vi "Ballard 1553 - Initialization VI.vi"(8 "error in (no error)":errorcluster, 10 "Custom XML":string, 11 "Device Item Ref in":T1 format="%.0x") -> (0 "error out":errorcluster, 3 "Device Item Ref out":T1 format="%.0x")   [LabVIEW 2017, in "Ballard 1553 System Explorer.lvlib"]
uses:
  Ballard 1553 System Explorer.lvlib
  <vilib>/NI Veristand/Custom Device API/Custom Device Item Ref.ctl
  <vilib>/NI Veristand/Custom Device API/Custom Device Channel.ctl
  <vilib>/NI Veristand/Custom Device API/Custom Device Channel Type.ctl
  Shared/Controls and Global/Initialization Method.ctl
  Shared/Controls and Global/Global.vi
  <vilib>/NI Veristand/Custom Device API/Set Item Property (U16).vi
  <vilib>/NI Veristand/Custom Device API/Set Item Property (I32).vi
  <vilib>/NI VeriStand/Custom Device API/Custom Device API.lvlib
  Shared/Ballard 1553 Shared.lvlib
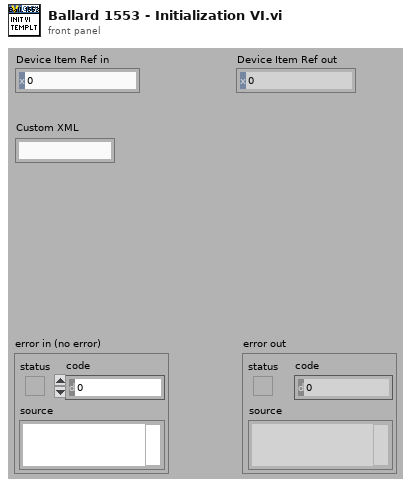
[diagram p1: front panel]
types:
  T1 = typedef "Custom Device API.lvlib/Custom Device Item Ref.ctl" = u64
  T2 = typedef "Ballard 1553 Shared.lvlib/Initialization Method.ctl" = enum16{"PXI Slot Number", "Card Number"}
  T3 = typedef "Custom Device API.lvlib/Custom Device Channel.ctl" = cluster{"Type":T4, "Units":string, "Default Value":dbl, "Faultable":bool, "Scalable":bool}
  T4 = typedef "Custom Device API.lvlib/Custom Device Channel Type.ctl" = enum16{"Input", "Output"}
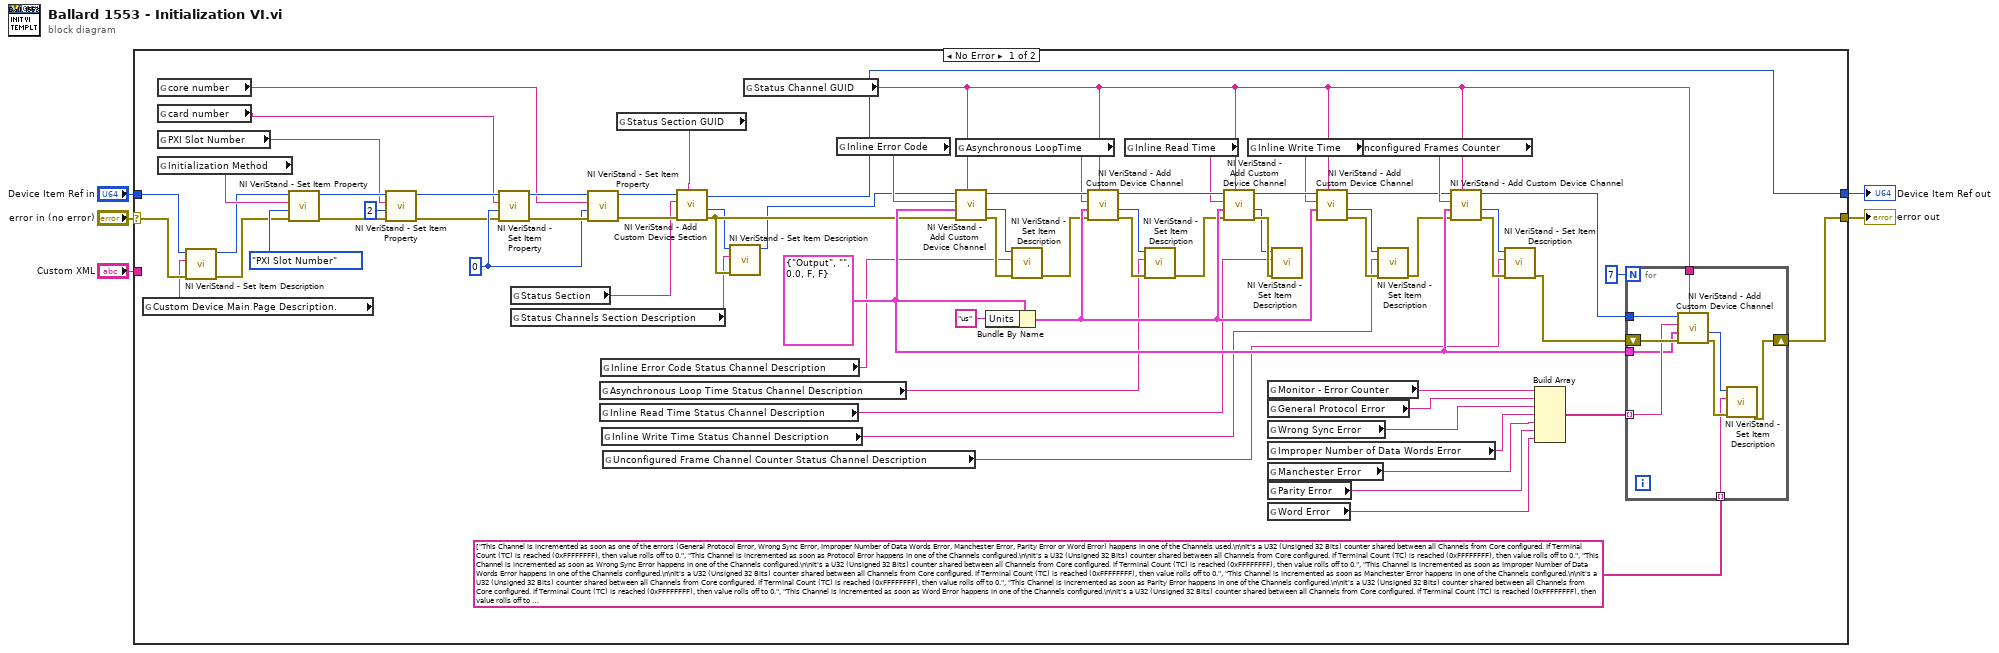
[diagram p0: block diagram]
diagram:
  n1 = case shown="No Error" "error in (no error)" {
    selector: "error in (no error)" -> [w12 w87]
    tunnel: [w75 w86] -> w4
    tunnel: "Device Item Ref in" -> [w14 w86]
    tunnel: "Custom XML" -> [_ _]
    tunnel: [w45 w87] -> w1
    frame No Error {
      w71 = 0 ("Value")
      w43 = T3 {"Type"=enum."Output", "Units"="", "Default Value"=0.0, "Faultable"=FALSE, "Scalable"=FALSE} ("Channel")
      n2 = global read "Global.vi" "Custom Device Main Page Description."() -> (w10:string)
      n3 = global read "Global.vi" "core number"() -> (w59:string)
      n4 = global read "Global.vi" "card number"() -> (w58:string)
      n5 = global read "Global.vi" "PXI Slot Number"() -> (w60:string)
      n6 = global read "Global.vi" "Initialization Method"() -> (w61:string)
      n7 = call <vilib>:"NI VeriStand - Set Item Description.vi"("error in (no error)"=w12, "Description"=w10, "Item Ref in"=w14) -> ("error out"=w11:errorcluster, "Item Ref out"=w13:T1)  [unwired: 6 in, 1 out]
      n8 = call-poly <vilib>:"NI VeriStand - Set Item Property.vi"("error in (no error)"=w11, "Value"=Initialization_Method."PXI Slot Number" ("Initialization Method"), "Property Name"=w61, "Item Ref in"=w13) -> ("error out"=w65:errorcluster, "Item Ref out"=w66:T1)  [unwired: 5 in, 1 out]
      n9 = call-poly <vilib>:"NI VeriStand - Set Item Property.vi"("error in (no error)"=w65, "Value"=2, "Property Name"=w60, "Item Ref in"=w66) -> ("error out"=w64:errorcluster, "Item Ref out"=w63:T1)  [unwired: 5 in, 1 out]
      n10 = call-poly <vilib>:"NI VeriStand - Set Item Property.vi"("error in (no error)"=w64, "Value"=w71, "Property Name"=w58, "Item Ref in"=w63) -> ("error out"=w72:errorcluster, "Item Ref out"=w73:T1)  [unwired: 5 in, 1 out]
      n11 = global read "Global.vi" "Status Section"() -> (w54:string)
      n12 = global read "Global.vi" "Status Channels Section Description"() -> (w6:string)
      n13 = call-poly <vilib>:"NI VeriStand - Set Item Property.vi"("error in (no error)"=w72, "Value"=w71, "Property Name"=w59, "Item Ref in"=w73) -> ("error out"=w57:errorcluster, "Item Ref out"=w56:T1)  [unwired: 5 in, 1 out]
      n14 = global read "Global.vi" "Asynchronous Loop Time Status Channel Description"() -> (w19:string)
      n15 = global read "Global.vi" "Inline Read Time Status Channel Description"() -> (w17:string)
      n16 = global read "Global.vi" "Inline Error Code Status Channel Description"() -> (w18:string)
      n17 = global read "Global.vi" "Inline Write Time Status Channel Description"() -> (w16:string)
      n18 = global read "Global.vi" "Unconfigured Frame Channel Counter Status Channel Description"() -> (w15:string)
      n19 = global read "Global.vi" "Status Section GUID"() -> (w55:string)
      n20 = call <vilib>:"NI VeriStand - Add Custom Device Section.vi"("GUID (Default Section)"=w55, "error in (no error)"=w57, "Section Name"=w54, "Parent Ref in"=w56) -> ("error out"=w9:errorcluster, "Section Ptr"=w8:T1, "Parent Ref out"=w75:T1)  [unwired: 4 in, 1 out]
      n21 = call <vilib>:"NI VeriStand - Set Item Description.vi"("error in (no error)"=w9, "Description"=w6, "Item Ref in"=w8) -> ("Item Ref out"=w7:T1)  [unwired: 6 in, 2 out]
      n22 = global read "Global.vi" "Status Channel GUID"() -> (w34:string)
      n23 = global read "Global.vi" "Inline Error Code"() -> (w53:string)
      n24 = global read "Global.vi" "Asynchronous LoopTime"() -> (w52:string)
      n25 = call <vilib>:"NI VeriStand - Add Custom Device Channel.vi"("GUID (Default Channel)"=w34, "error in (no error)"=w9, "Channel"=w43, "Channel Name"=w53, "Parent Ref in"=w7) -> ("error out"=w33:errorcluster, "Channel Ref"=w24:T1, "Parent Ref out"=w68:T1)  [unwired: 3 in, 1 out]
      n26 = Bundle By Name(cluster=w43, "Units"="us") -> (w69:T3)
      n27 = call <vilib>:"NI VeriStand - Set Item Description.vi"("error in (no error)"=w33, "Description"=w18, "Item Ref in"=w24) -> ("error out"=w25:errorcluster)  [unwired: 6 in, 2 out]
      n28 = call <vilib>:"NI VeriStand - Add Custom Device Channel.vi"("GUID (Default Channel)"=w34, "error in (no error)"=w25, "Channel"=w69, "Channel Name"=w52, "Parent Ref in"=w68) -> ("error out"=w32:errorcluster, "Channel Ref"=w23:T1, "Parent Ref out"=w76:T1)  [unwired: 3 in, 1 out]
      n29 = global read "Global.vi" "Inline Read Time"() -> (w51:string)
      n30 = call <vilib>:"NI VeriStand - Set Item Description.vi"("error in (no error)"=w32, "Description"=w19, "Item Ref in"=w23) -> ("error out"=w26:errorcluster)  [unwired: 6 in, 2 out]
      n31 = call <vilib>:"NI VeriStand - Add Custom Device Channel.vi"("GUID (Default Channel)"=w34, "error in (no error)"=w26, "Channel"=w69, "Channel Name"=w51, "Parent Ref in"=w76) -> ("error out"=w31:errorcluster, "Channel Ref"=w22:T1, "Parent Ref out"=w70:T1)  [unwired: 3 in, 1 out]
      n32 = global read "Global.vi" "Inline Write Time"() -> (w50:string)
      n33 = global read "Global.vi" "Monitor - Error Counter"() -> (w41:string)
      n34 = global read "Global.vi" "General Protocol Error"() -> (w40:string)
      n35 = global read "Global.vi" "Wrong Sync Error"() -> (w39:string)
      n36 = global read "Global.vi" "Improper Number of Data Words Error"() -> (w38:string)
      n37 = global read "Global.vi" "Manchester Error"() -> (w37:string)
      n38 = global read "Global.vi" "Parity Error"() -> (w36:string)
      n39 = global read "Global.vi" "Word Error"() -> (w35:string)
      n40 = call <vilib>:"NI VeriStand - Set Item Description.vi"("error in (no error)"=w31, "Description"=w17, "Item Ref in"=w22) -> ()  [unwired: 6 in, 3 out]
      n41 = call <vilib>:"NI VeriStand - Add Custom Device Channel.vi"("GUID (Default Channel)"=w34, "Channel"=w69, "Channel Name"=w50, "Parent Ref in"=w70) -> ("error out"=w30:errorcluster, "Channel Ref"=w21:T1, "Parent Ref out"=w48:T1)  [unwired: 4 in, 1 out]
      n42 = global read "Global.vi" "Unconfigured Frames Counter"() -> (w49:string)
      n43 = call <vilib>:"NI VeriStand - Set Item Description.vi"("error in (no error)"=w30, "Description"=w16, "Item Ref in"=w21) -> ("error out"=w27:errorcluster)  [unwired: 6 in, 2 out]
      n44 = call <vilib>:"NI VeriStand - Add Custom Device Channel.vi"("GUID (Default Channel)"=w34, "error in (no error)"=w27, "Channel"=w43, "Channel Name"=w49, "Parent Ref in"=w48) -> ("error out"=w29:errorcluster, "Channel Ref"=w20:T1, "Parent Ref out"=w42:T1)  [unwired: 3 in, 1 out]
      n45 = call <vilib>:"NI VeriStand - Set Item Description.vi"("error in (no error)"=w29, "Description"=w15, "Item Ref in"=w20) -> ("error out"=w28:errorcluster)  [unwired: 6 in, 2 out]
      n46 = Build Array(w41, w40, w39, w38, w37, w36, w35) -> (w44:string[])
      n47 = for {
        N: 7 -> [_]
        tunnel: string[] ["This Channel is incremented as soon as one of the errors (General Protocol Error, Wrong Sync Error, Improper Number of Data Words Error, Manchester Error, Parity Error or Word Error) happens in one of the Channels used.\n\nIt's a U32 (Unsigned 32 Bits) counter shared between all Channels from Core configured. If Terminal Count (TC) is reached (0xFFFFFFFF), then value rolls off to 0.", "This Channel is incremented as soon as Protocol Error happens in one of the Channels configured.\n\nIt's a U32 (Unsigned 32 Bits) counter shared between all Channels from Core configured. If Terminal Count (TC) is reached (0xFFFFFFFF), then value rolls off to 0.", "This Channel is incremented as soon as Wrong Sync Error happens in one of the Channels configured.\n\nIt's a U32 (Unsigned 32 Bits) counter shared between all Channels from Core configured. If Terminal Count (TC) is reached (0xFFFFFFFF), then value rolls off to 0.", "This Channel is incremented as soon as Improper Number of Data Words Error happens in one of the Channels configured.\n\nIt's a U32 (Unsigned 32 Bits) counter shared between all Channels from Core configured. If Terminal Count (TC) is reached (0xFFFFFFFF), then value rolls off to 0.", "This Channel is incremented as soon as Manchester Error happens in one of the Channels configured.\n\nIt's a U32 (Unsigned 32 Bits) counter shared between all Channels from Core configured. If Terminal Count (TC) is reached (0xFFFFFFFF), then value rolls off to 0.", "This Channel is incremented as soon as Parity Error happens in one of the Channels configured.\n\nIt's a U32 (Unsigned 32 Bits) counter shared between all Channels from Core configured. If Terminal Count (TC) is reached (0xFFFFFFFF), then value rolls off to 0.", "This Channel is incremented as soon as Word Error happens in one of the Channels configured.\n\nIt's a U32 (Unsigned 32 Bits) counter shared between all Channels from Core configured. If Terminal Count (TC) is reached (0xFFFFFFFF), then value rolls off to 0."] -> [w83] mode=indexing
        shift-right: [w81] -> w45
        shift-left: w28 -> [w82]
        tunnel: w44 -> [w80] mode=indexing
        tunnel: w43 -> [w79]
        tunnel: w42 -> [w78]
        tunnel: w34 -> [w77]
        n48 = call <vilib>:"NI VeriStand - Add Custom Device Channel.vi"("GUID (Default Channel)"=w77, "error in (no error)"=w82, "Channel"=w79, "Channel Name"=w80, "Parent Ref in"=w78) -> ("error out"=w85:errorcluster, "Channel Ref"=w84:T1)  [unwired: 3 in, 2 out]
        n49 = call <vilib>:"NI VeriStand - Set Item Description.vi"("error in (no error)"=w85, "Description"=w83, "Item Ref in"=w84) -> ("error out"=w81:errorcluster)  [unwired: 6 in, 2 out]
      }
    }
    frame Error {
    }
  }
  "error out" <- w1
  "Device Item Ref out" <- w4
